vi "sns topic sample.vi"() -> ()   [LabVIEW 2015]
uses:
  Topic/Topic Attribute Value Pair.ctl
  Topic/Topic Attribute.ctl
  Topic/Topic.lvclass
  Core/HTTP Request/AWS Credentials.ctl
  Core/HTTP Request/Region.ctl
  Topic/Mutable Topic Attribute Value Pair.ctl
  Topic/Mutable Topic Attribute.ctl
  Core/HTTP Request/HTTP Request.lvclass
panel:
  out "error out":errorcluster
  out "Topics out":refnum<class "Topic.lvclass">[](array[class])
  out "Topic Attribute Value Pairs 2":T1[](array[typedef])
  out "Topic Attribute Value Pairs":T1[](array[typedef])
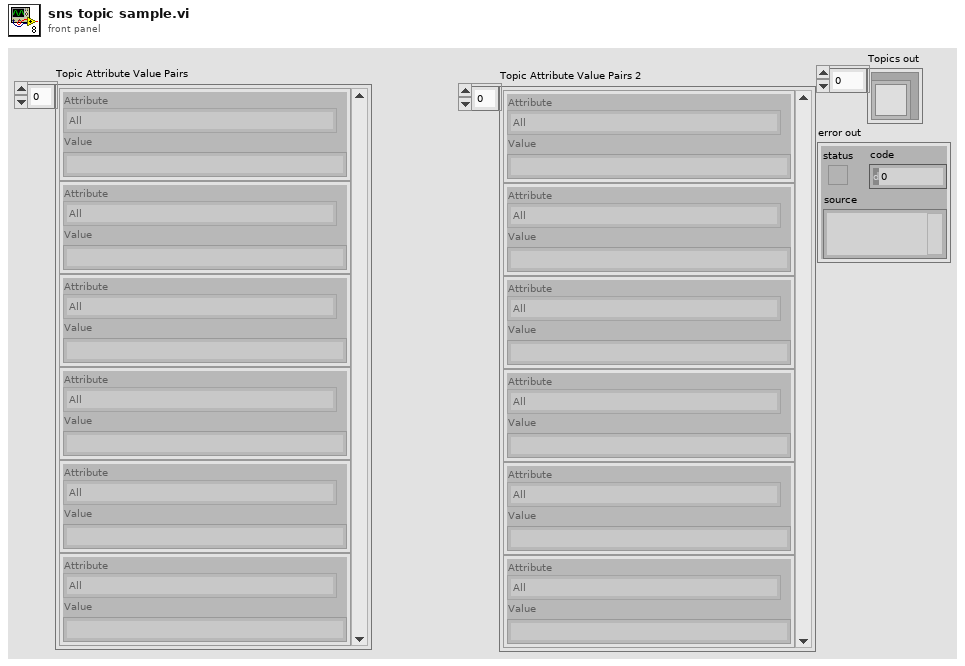
[diagram p1: front panel]
types:
  T1 = typedef "NI_AWS_SNS.lvlib/Topic.lvclass/Topic Attribute Value Pair.ctl" = cluster{"Attribute":T2, "Value":string}
  T2 = typedef "NI_AWS_SNS.lvlib/Topic.lvclass/Topic Attribute.ctl" = enum16{"All", "TopicArn", "Owner", "Policy", "DisplayName", "SubscriptionsPending", "SubscriptionsConfirmed", "SubscriptionsDeleted", "DeliveryPolicy", "EffectiveDeliveryPolicy"}
  T3 = typedef "NI_AWS_SNS.lvlib/Topic.lvclass/Mutable Topic Attribute Value Pair.ctl" = cluster{"Attribute":T4, "Value":string}
  T4 = typedef "NI_AWS_SNS.lvlib/Topic.lvclass/Mutable Topic Attribute.ctl" = enum16{"Policy", "DisplayName", "DeliveryPolicy"}
  T5 = typedef "NI_AWS_Core.lvlib/HTTP Request.lvclass/Region.ctl" = enum16{"us-east-1", "us-east-2", "us-west-1", "us-west-2", "ap-northeast-1", "ap-northeast-2", "ap-southeast-1", "ap-southeast-2", "ca-central-1", "eu-central-1", "eu-west-1", "eu-west-2", "sa-east-1"}
  T6 = typedef "NI_AWS_Core.lvlib/HTTP Request.lvclass/AWS Credentials.ctl" = cluster{"Access Key":string, "Secret Key":string}
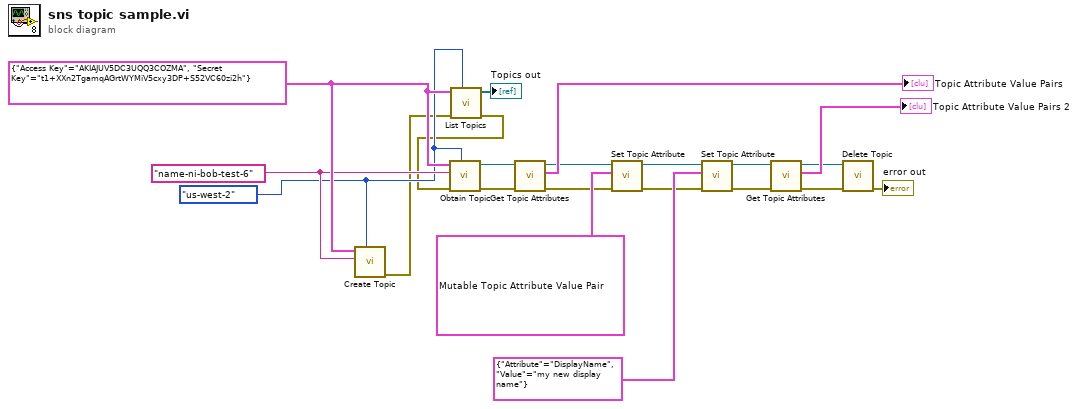
[diagram p0: block diagram]
diagram:
  w9 = Region."us-west-2" ("Region")
  w12 = T6 {"Access Key"="AKIAJUV5DC3UQQ3COZMA", "Secret Key"="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"} ("AWS Credentials")
  w11 = "name-ni-bob-test-6" ("Name")
  n1 = call "Create Topic.vi"("Region"=w9, "Name"=w11, "AWS Credentials"=w12) -> ("error out"=w8:errorcluster)  [unwired: 7 in, 1 out]
  n2 = call "List Topics.vi"("Region"=w9, "error in (no error)"=w8, "AWS Credentials"=w12) -> ("error out"=w7:errorcluster, "Topics out"=→"Topics out":refnum<class "Topic.lvclass">[])  [unwired: 7 in]
  n3 = call "Obtain Topic.vi"("Region"=w9, "error in (no error)"=w7, "Name"=w11, "AWS Credentials"=w12) -> ("error out"=w6:errorcluster, "Topic out"=w21:refnum<class "Topic.lvclass">)  [unwired: 5 in, 1 out]
  n4 = call "Get Topic Attributes.vi"("error in (no error)"=w6, "Topic"=w21) -> ("error out"=w5:errorcluster, "Topic Attributes"=→"Topic Attribute Value Pairs":T1[], "Topic out"=w19:refnum<class "Topic.lvclass">)  [unwired: 7 in]
  n5 = call "Set Topic Attribute.vi"("error in (no error)"=w5, "Topic Attribute"=T3 {"Attribute"=enum."Policy", "Value"="{\n  \"Version\": \"2008-10-17\",\n  \"Id\": \"__default_policy_ID\",\n  \"Statement\": [\n    {\n      \"Sid\": \"__default_statement_ID\",\n      \"Effect\": \"Allow\",\n      \"Principal\": {\n        \"AWS\": \"*\"\n      },\n      \"Action\": [\n        \"SNS:Publish\",\n        \"SNS:RemovePermission\",\n        \"SNS:SetTopicAttributes\",\n        \"SNS:DeleteTopic\",\n        \"SNS:ListSubscriptionsByTopic\",\n        \"SNS:GetTopicAttributes\",\n        \"SNS:Receive\",\n        \"SNS:AddPermission\",\n        \"SNS:Subscribe\"\n      ],\n      \"Resource\": \"arn:aws:sns:us-west-2:143260871048:dnatt-test-sns-topic\",\n      \"Condition\": {\n        \"StringEquals\": {\n          \"AWS:SourceOwner\": \"143260871048\"\n        }\n      }\n    },\n    {\n      \"Sid\": \"__console_pub_0\",\n      \"Effect\": \"Allow\",\n      \"Principal\": {\n        \"AWS\": \"*\"\n      },\n      \"Action\": \"SNS:Publish\",\n      \"Resource\": \"arn:aws:sns:us-west-2:143260871048:dnatt-test-sns-topic\"\n    },\n    {\n      \"Sid\": \"__console_sub_0\",\n      \"Effect\": \"Allow\",\n      \"Principal\": {\n        \"AWS\": \"*\"\n      },\n      \"Action\": [\n        \"SNS:Subscribe\",\n        \"SNS:Receive\"\n      ],\n      \"Resource\": \"arn:aws:sns:us-west-2:143260871048:dnatt-test-sns-topic\"\n    }\n  ]\n}"} ("Topic Attribute Value Pair"), "Topic"=w19) -> ("error out"=w4:errorcluster, "Topic out"=w17:refnum<class "Topic.lvclass">)  [unwired: 7 in]
  n6 = call "Set Topic Attribute.vi"("error in (no error)"=w4, "Topic Attribute"=T3 {"Attribute"=enum."DisplayName", "Value"="my new display name"} ("Topic Attribute Value Pair"), "Topic"=w17) -> ("error out"=w3:errorcluster, "Topic out"=w15:refnum<class "Topic.lvclass">)  [unwired: 7 in]
  n7 = call "Get Topic Attributes.vi"("error in (no error)"=w3, "Topic"=w15) -> ("error out"=w2:errorcluster, "Topic Attributes"=→"Topic Attribute Value Pairs 2":T1[], "Topic out"=w13:refnum<class "Topic.lvclass">)  [unwired: 7 in]
  n8 = call "Delete Topic.vi"("error in (no error)"=w2, "Topic"=w13) -> ("error out"=→"error out":errorcluster)  [unwired: 9 in]
